vi "UpdateState2.vi"(0 "XRef":T14, 1 "Old State":T13, 2 "Version":T11) -> (14 "Is Good?":T10, 15 "Reply":T8, 17 "State Out":T1 {"BlockNodeState"."Draw Style" items=["FunctionBlock", "ExpressVI", "Variable", "Elemental I/O", "32x32 Icon", "FunctionBlockCompact"]; "BlockNodeState"."Terminal Data"."Terminal Flags" format="%.0b"})   [LabVIEW 2017, in "ExpressFormulaBlockNode.xnode"]
uses:
  <vilib>/express/express arith-compare/Formula/XNode/ExpressFormulaBlockNode.xnode
  <vilib>/XNodeSupport/XNodeXNodeRef.ctl
  <vilib>/XNodeSupport/XNodeVariant.ctl
  <vilib>/XNodeSupport/XNodeVersion.ctl
  <vilib>/XNodeSupport/XNodeUShort.ctl
  <vilib>/XNodeSupport/XNodeBool.ctl
  <vilib>/XNodeSupport/XNodeStringArray.ctl
  <vilib>/XNodeSupport/XNodeString.ctl
  <vilib>/express/express arith-compare/Formula/XNode/State.ctl
  <vilib>/BlockNodeSupport/BlockNodeState.ctl
  <vilib>/BlockNodeSupport/TerminalData.ctl
  <vilib>/picture/picture.llb/imagedata.ctl
  <vilib>/express/express shared/XNodes/controls/ExpressState.ctl
  <vilib>/express/express shared/XNodes/controls/ExpressTerminalInfo.ctl
  <vilib>/XNodeSupport/XNodeType.ctl
  <vilib>/XNodeSupport/NI_XNodeSupport.lvlib
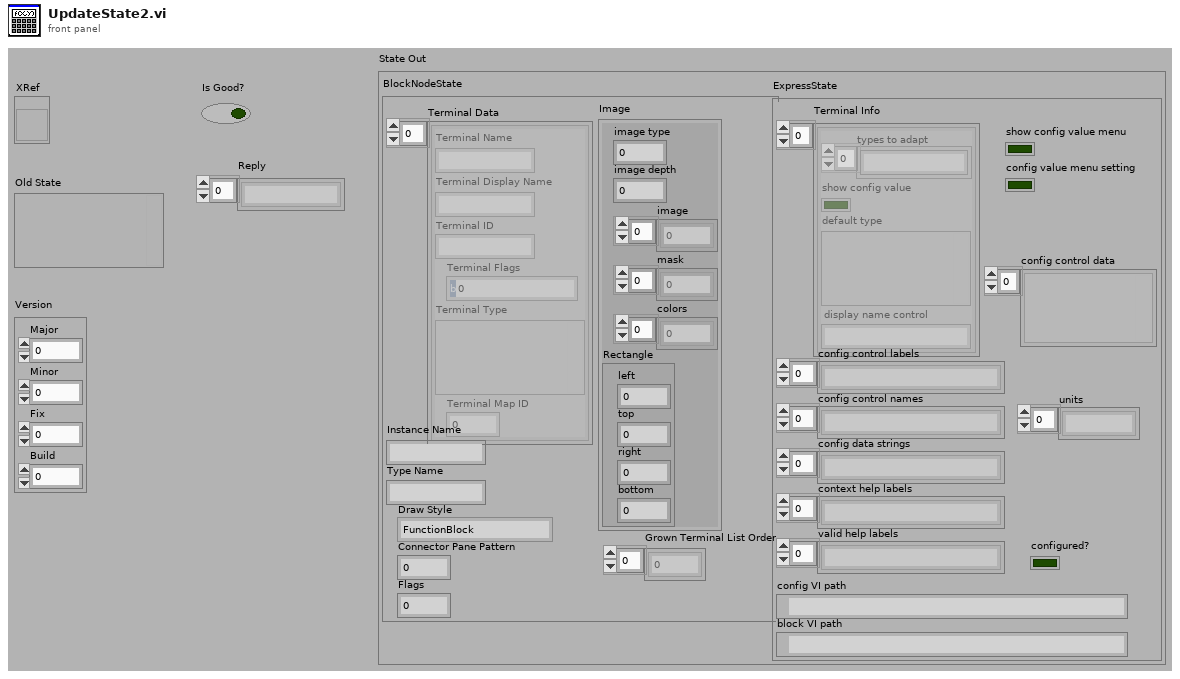
[diagram p1: front panel]
types:
  T1 = typedef "ExpressFormulaBlockNode.xnode/State.ctl" = cluster{"BlockNodeState":T2, "ExpressState":T5}
  T2 = typedef "BlockNodeState.ctl" = cluster{"Terminal Data":T3[], "Instance Name":string, "Type Name":string, "Draw Style":i32, "Connector Pane Pattern":i32, "Flags":i32, "Grown Terminal List Order":i32[], "Image":T4}
  T3 = typedef "TerminalData.ctl" = cluster{"Terminal Name":string, "Terminal Display Name":string, "Terminal ID":string, "Terminal Flags":i32, "Terminal Type":variant, "Terminal Map ID":i32}
  T4 = typedef "imagedata.ctl" = cluster{"image type":i32, "image depth":i32, "image":u8[], "mask":u8[], "colors":u32[], "Rectangle":cluster{"left":i16, "top":i16, "right":i16, "bottom":i16}}
  T5 = typedef "ExpressState.ctl" = cluster{"Terminal Info":T6, "config control names":string[], "config data strings":string[], "config control data":variant[], "units":string[], "configured?":bool, "config VI path":path, "block VI path":path, "config control labels":string[], "show config value menu":bool, "config value menu setting":bool, "context help labels":string[], "valid help labels":string[]}
  T6 = typedef "ExpressTerminalInfo.ctl" = cluster{"types to adapt":string[], "show config value":bool, "default type":T7, "display name control":string}[]
  T7 = typedef "NI_XNodeSupport.lvlib/XNodeType.ctl" = variant
  T8 = typedef "NI_XNodeSupport.lvlib/XNodeStringArray.ctl" = T9[]
  T9 = typedef "NI_XNodeSupport.lvlib/XNodeString.ctl" = string
  T10 = typedef "NI_XNodeSupport.lvlib/XNodeBool.ctl" = bool
  T11 = typedef "NI_XNodeSupport.lvlib/XNodeVersion.ctl" = cluster{"Major":T12, "Minor":T12, "Fix":T12, "Build":T12}
  T12 = typedef "NI_XNodeSupport.lvlib/XNodeUShort.ctl" = u16
  T13 = typedef "NI_XNodeSupport.lvlib/XNodeVariant.ctl" = variant
  T14 = typedef "NI_XNodeSupport.lvlib/XNodeXNodeRef.ctl" = refnum<vi>
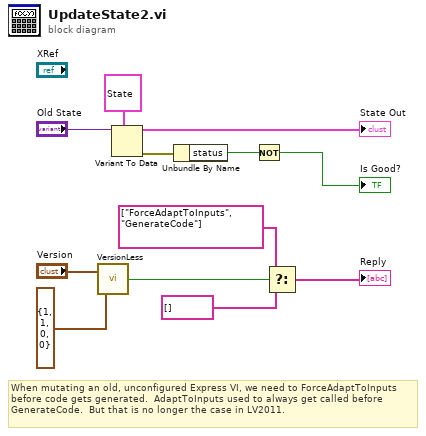
[diagram p0: block diagram]
diagram:
  # "When mutating an old, unconfigured Express VI, we need to ForceAdaptToInputs before code gets generated.  AdaptToInputs used to always get called before GenerateCode.  But that is no longer the case in LV2011."
  n1 = call <vilib>:"VersionLess.vi"("y"=T11 {"Major"=1, "Minor"=1, "Fix"=0, "Build"=0} ("Version"), "x"="Version") -> ("x < y?"=w5:bool)
  n2 = Variant To Data(type=T1 {"BlockNodeState"={"Terminal Data"=[], "Instance Name"="", "Type Name"="", "Draw Style"=0, "Connector Pane Pattern"=0, "Flags"=0, "Grown Terminal List Order"=[], "Image"={"image type"=0, "image depth"=0, "image"=[], "mask"=[], "colors"=[], "Rectangle"={"left"=0, "top"=0, "right"=0, "bottom"=0}}}, "ExpressState"={"Terminal Info"=[], "config control names"=[], "config data strings"=[], "config control data"=[], "units"=[], "configured?"=FALSE, "config VI path"=path "", "block VI path"=path "", "config control labels"=[], "show config value menu"=FALSE, "config value menu setting"=FALSE, "context help labels"=[], "valid help labels"=[]}} ("State Out"), Variant="Old State") -> (data=→"State Out":T1, error out=w9:errorcluster)  [unwired: 1 in]
  n3 = Unbundle By Name(w9) -> ("status"=w8:bool)
  n4 = Not(x=w8) -> (.not. x?=→"Is Good?":bool)
  n5 = Select(t=T8 ["ForceAdaptToInputs", "GenerateCode"] ("Reply"), s=w5, f=T8 [] ("Reply")) -> (s? t:f=→"Reply":T8)
